vi "SequenceAcquisition.vi"() -> ()   [LabVIEW 2018]
uses:
  C:/Users/Public/Documents/Photometrics/PMQI-LabViewSamples/Examples/Dependencies/PVCamNET.dll
  Public/Documents/Photometrics/PMQI-LabViewSamples/Examples/Dependencies/PVCamNET.dll
panel:
  out "Capturing":bool
  in  "?":bool
  in  "?":bool
  in  "Exposure":u32
  in  "FramesToCapture":u16
  # "SequenceAcqusition.vi\n\nDescription:\nThis sample code lets the user use sequence mode with \nthe user's preferred buffer size (framesToCapture) and exposure time. \n\nSteps to run:\n1. Click \"Run\"\n2. Enter FramesToCapture and Exposure time\n3. Click \"START\"\n4. Click \"STOP\""
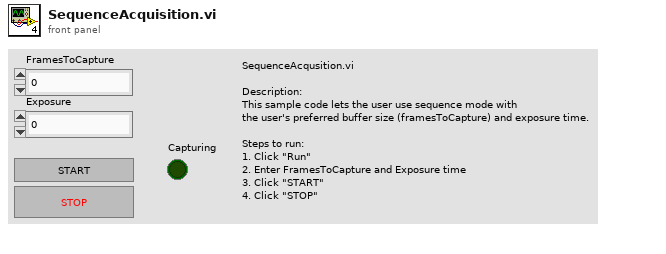
[diagram p1: front panel]
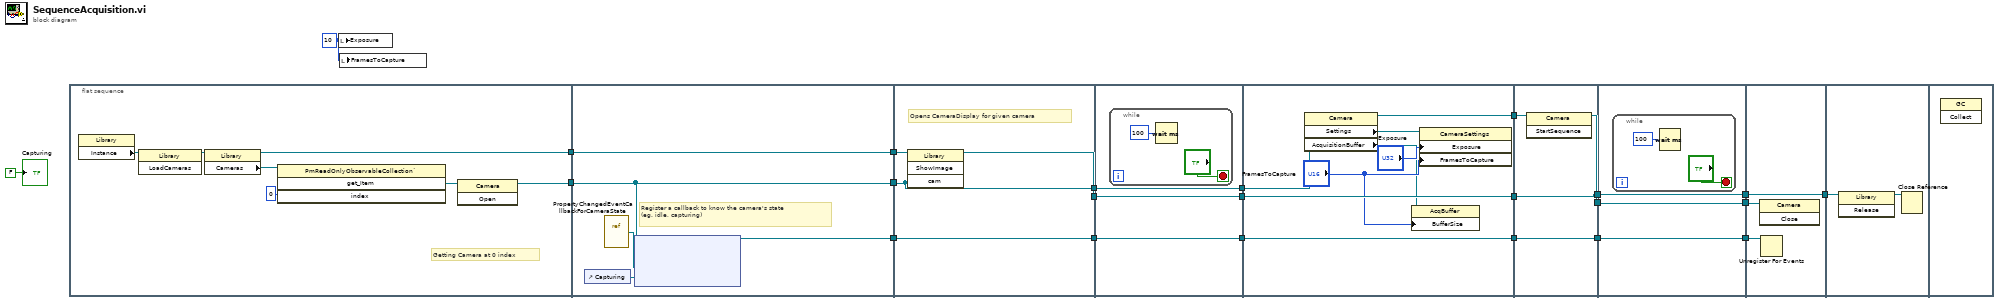
[diagram p0: block diagram]
diagram:
  w1 = u32 10 ("Exposure")
  n1 = flat-sequence {
    tunnel: [w26] -> w12
    tunnel: [w27] -> w10
    tunnel: w12 -> [w35]
    tunnel: [w35] -> w11
    tunnel: w10 -> [w32]
    tunnel: [w32] -> w9
    tunnel: [w31] -> w3
    tunnel: w11 -> [w39]
    tunnel: w9 -> [w38]
    tunnel: [w38] -> w22
    tunnel: [w37] -> w23
    tunnel: [w36] -> w4
    tunnel: w3 -> [w36]
    tunnel: w23 -> [w42]
    tunnel: [w42] -> w21
    tunnel: w22 -> [w41]
    tunnel: [w41] -> w20
    tunnel: [w40] -> w5
    tunnel: w4 -> [w40]
    tunnel: [w52] -> w19
    tunnel: [w51] -> w18
    tunnel: w21 -> [w51]
    tunnel: w20 -> [w50]
    tunnel: [w47] -> w6
    tunnel: w5 -> [w47]
    tunnel: w19 -> [w54]
    tunnel: [w53] -> w16
    tunnel: w18 -> [w56]
    tunnel: [w56] -> w14
    tunnel: [w55] -> w7
    tunnel: w6 -> [w55]
    tunnel: w16 -> [w59]
    tunnel: [w59] -> w15
    tunnel: w14 -> [w58]
    tunnel: [w58] -> w13
    tunnel: w7 -> [w57]
    tunnel: [w57] -> w2
    tunnel: w15 -> [w64]
    tunnel: w13 -> [w63]
    tunnel: [w63] -> w17
    tunnel: w2 -> [w62]
    tunnel: w17 -> [w66]
    frame #0 {
      # "Getting Camera at 0 index"
      n2 = property class="Library"() -> ("Instance"=w25:refnum<k24>)  [unwired: 2 in, 2 out]
      n3 = invoke class="Library" method="LoadCameras"(reference=w25) -> (reference out=w24:refnum<k24>)  [unwired: 2 in, 2 out]
      n4 = property class="Library"(reference=w24) -> (reference out=w26:refnum<k24>, "Cameras"=w30:refnum<k24>)  [unwired: 1 in, 1 out]
      n5 = invoke class="PmReadOnlyObservableCollection`" method="get_Item"(reference=w30, "index"=0) -> ("get_Item"=w28:refnum<k24>)  [unwired: 2 in, 3 out]
      n6 = invoke class="Camera" method="Open"(reference=w28) -> (reference out=w27:refnum<k24>)  [unwired: 2 in, 2 out]
    }
    frame #1 {
      # "Register a callback to know the camera's state \n(eg. idle, capturing)"
      n7 = control-ref of="Capturing"() -> (w34:refnum<vi>)
      n8 = vi-ref "PropertyChangedEventCallbackForCameraState.vi"() -> ("vi reference"=w33:refnum<vi>)
      n9 = node(w32, w33, w34) -> (w31:refnum<k27>)  [unwired: 2 in, 1 out]
    }
    frame #2 {
      # "Opens CameraDisplay for given camera"
      n10 = invoke class="Library" method="ShowImage"(reference=w39, "cam"=w38) -> (reference out=w37:refnum<k24>)  [unwired: 2 in, 3 out]
    }
    frame #3 {
      n11 = while {
        stop <- "?" stop-if-true
        n12 = Wait (ms)(milliseconds to wait=u32 100) -> ()  [unwired: 1 out]
      }
    }
    frame #4 {
      n13 = property class="Camera"(reference=w50) -> (reference out=w52:refnum<k24>, "Settings"=w49:refnum<k24>, "AcquisitionBuffer"=w45:refnum<k24>)  [unwired: 1 in, 1 out]
      n14 = property class="AcqBuffer"(reference=w45, "BufferSize"="FramesToCapture") -> ()  [unwired: 1 in, 2 out]
      n15 = property class="CameraSettings"(reference=w49, "Exposure"="Exposure", "FramesToCapture"="FramesToCapture") -> ()  [unwired: 1 in, 2 out]
    }
    frame #5 {
      n16 = invoke class="Camera" method="StartSequence"(reference=w54) -> (reference out=w53:refnum<k24>)  [unwired: 2 in, 2 out]
    }
    frame #6 {
      n17 = while {
        stop <- "?" stop-if-true
        n18 = Wait (ms)(milliseconds to wait=u32 100) -> ()  [unwired: 1 out]
      }
    }
    frame #7 {
      n19 = invoke class="Camera" method="Close"(reference=w64) -> ()  [unwired: 2 in, 3 out]
      n20 = Unregister For Events(event registration refnum=w62) -> ()  [unwired: 1 in, 1 out]
    }
    frame #8 {
      n21 = invoke class="Library" method="Release"(reference=w66) -> (reference out=w65:refnum<k24>)  [unwired: 2 in, 2 out]
      n22 = Close Reference(reference=w65) -> ()  [unwired: 1 in, 1 out]
    }
    frame #9 {
      n23 = invoke class="GC" method="Collect"() -> ()  [unwired: 3 in, 3 out]
    }
  }
  n24 = local write "Exposure"(w1) -> ()
  n25 = local write "FramesToCapture"(w1) -> ()
  "Capturing" <- FALSE ("Capturing")
